vi "Init Refs.vi"(10 "Refs":T1) -> (3 "TEMPLATE Refs out":refnum<class "TEMPLATE Refs.lvclass">)   [LabVIEW 2025, in "_Template.lvlib" / "Templates.lvlib" / "TEMPLATE Actor.lvlib" / "TEMPLATE Refs.lvclass"]
uses:
  TEMPLATE Refs.lvclass
  Refs.ctl
  TEMPLATE Refs.lvclass/TEMPLATE Refs.ctl
  TEMPLATE Actor.lvlib
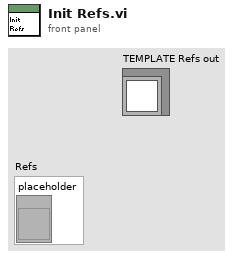
[diagram p1: front panel]
types:
  T1 = typedef "_Template.lvlib/Templates.lvlib/TEMPLATE Actor.lvlib/Refs.ctl" = cluster{"placeholder":refnum<vi>}
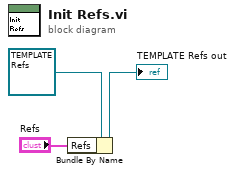
[diagram p0: block diagram]
diagram:
  n1 = Bundle By Name(cluster=refnum<class "TEMPLATE Refs.lvclass"> refnum ("TEMPLATE Refs out"), "Refs"="Refs") -> (→"TEMPLATE Refs out":refnum<class "TEMPLATE Refs.lvclass">)
